vi "송신vi.vi"() -> ()   [LabVIEW 2014]
panel:
  in  "정지":bool
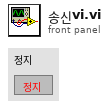
[diagram p1: front panel]
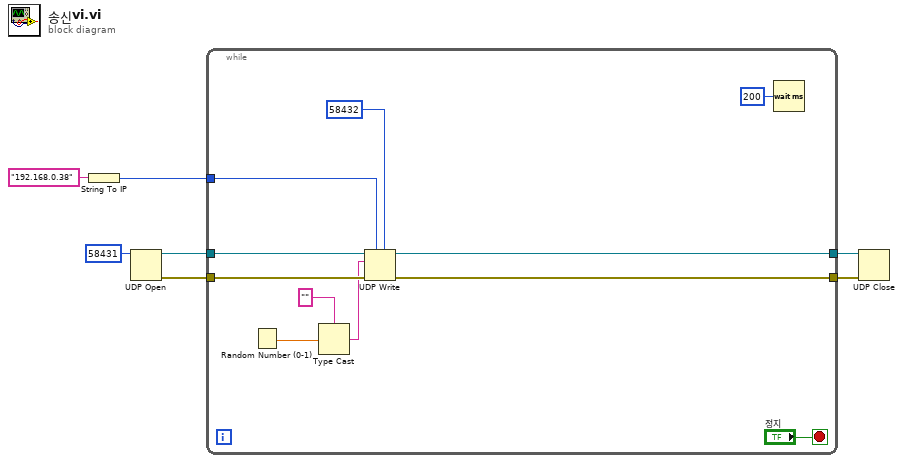
[diagram p0: block diagram]
diagram:
  n1 = String To IP(1:"192.168.0.38") -> (0:w1:u32)
  n2 = UDP Open(11:u16 58431 ("포트")) -> (port=w7:refnum<k16>, 0:w6:errorcluster)  [unwired: 4 in, 1 out]
  n3 = while {
    tunnel: w7 -> [w18]
    tunnel: w6 -> [w17]
    tunnel: [w16] -> w5
    tunnel: [w15] -> w4
    tunnel: w1 -> [w13]
    stop <- "정지" stop-if-true
    n4 = Random Number (0-1)() -> (number: 0 to 1=w10:dbl)
    n5 = Type Cast(type="" ("타입"), x=w10) -> (*(type *) &x=w9:string)
    n6 = UDP Write(address=w13, port or service name=u16 58432 ("포트 또는 서비스 이름"), connection ID=w18, data in=w9, 8:w17) -> (error out=w15:errorcluster, 3:w16:refnum<k16>)  [unwired: 1 in]
    n7 = Wait (ms)(milliseconds to wait=u32 200 ("대기 시간(ms)")) -> ()  [unwired: 1 out]
  }
  n8 = UDP Close(connection ID=w5, 8:w4) -> ()  [unwired: 2 out]
